vi "Get RT Index from Label and SDI in Word.vi"(11 "word in":u32 format="%032b") -> (1 "label index":i32 format="%0d", 3 "word out":u32 format="%032b", 5 "SDI":u32 format="%0d", 7 "label":u32)   [LabVIEW 2020, in "Ballard ARINC 429 Engine.lvlib" / "Custom Device.lvlib"]
uses:
  Custom Device.lvlib
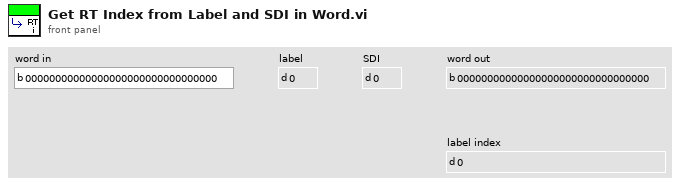
[diagram p1: front panel]
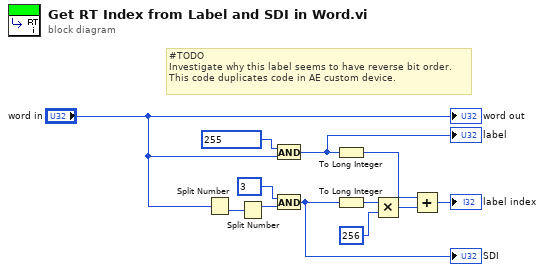
[diagram p0: block diagram]
diagram:
  # "#TODO\nInvestigate why this label seems to have reverse bit order.\nThis code duplicates code in AE custom device."
  n1 = Split Number(x="word in") -> (lo(x)=w10:u16)  [unwired: 1 out]
  n2 = Split Number(x=w10) -> (hi(x)=w11:u8)  [unwired: 1 out]
  n3 = And(x=u32 255 ("y"), y="word in") -> (x .and. y?=w4:u32)
  "label" <- w4
  n4 = And(x=u8 3, y=w11) -> (x .and. y?=w1:u8)
  "SDI" <- w1
  n5 = To Long Integer(number=w4) -> (32bit integer=w9:i32)
  n6 = To Long Integer(number=w1) -> (32bit integer=w5:i32)
  n7 = Multiply(x=w5, y=256) -> (x*y=w6:i32)
  n8 = Add(x=w9, y=w6) -> (x+y=→"label index":i32)
  "word out" <- "word in"
